vi "Keithley Log Ramp 3940 Amp.vi"(2 "Point #":i32, 3 "GPIB Data In":dbl[](array[numeric]) format="%.2e", 4 "Parameters":dbl[](array[numeric]) format="%.3e", 5 "VISA session":refnum<visa-resource-name>) -> (0 "Stop":bool, 1 "Keithley 3940 Voltage":dbl[](array[numeric]) format="%.3e")   [LabVIEW 2025]
doc: "Author: Scott Hannahs <sth@magnet.fsu.edu>\n\nThis software is licensed for use under the “MIT License\"\nCopyright (c) 2025 Scott Hannahs, sth@sth@magnet.sthnet.net\n\nPermission is hereby granted, free of charge, to any person obtaining a copy of this software and associated documentation files (the \"Software\"), to deal in the Software without restriction, including without limitation the rights to use, copy, modify, merge, publish, distribute, sublicense, and/or sell copies of the Software, and to permit persons to whom the Software is furnished to do so, subject to the following conditions: The above copyright notice and this permission notice shall be included in all copies or substantial portions of the Software.\n\nTHE SOFTWARE IS PROVIDED \"AS IS\", WITHOUT WARRANTY OF ANY KIND, EXPRESS OR IMPLIED, INCLUDING BUT NOT LIMITED TO THE WARRANTIES OF MERCHANTABILITY, FITNESS FOR A PARTICULAR PURPOSE AND NONINFRINGEMENT. IN NO EVENT SHALL THE AUTHORS OR COPYRIGHT HOLDERS BE LIABLE FOR ANY CLAIM, DAMAGES OR OTHER LIABILITY, WHETHER IN AN ACTION OF CONTRACT, TORT OR OTHERWISE, ARISING FROM, OUT OF OR IN CONNECTION WITH THE SOFTWARE OR THE USE OR OTHER DEALINGS IN THE SOFTWARE."
panel:
  out "I0":dbl format="%.3e"
  out "I":dbl format="%.3e"
  out "Delta":dbl format="%.2f"
  # "# pts/decade"
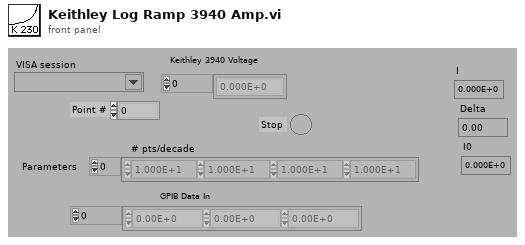
[diagram p1: front panel]
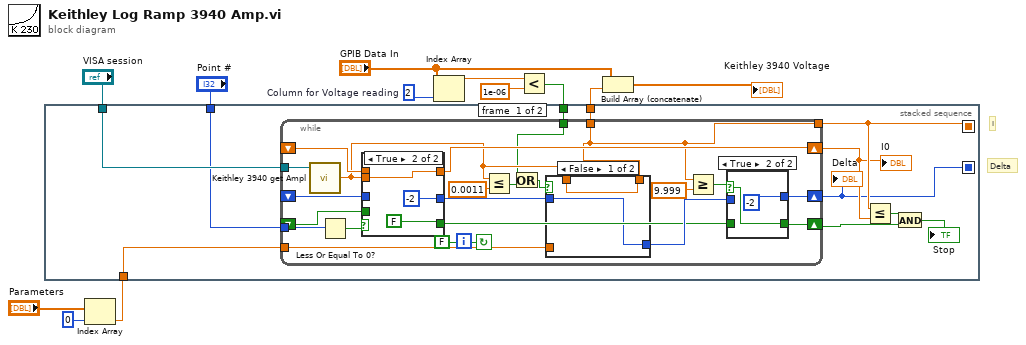
[diagram p0: block diagram]
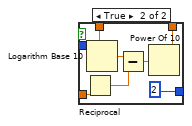
[diagram p3: hidden frame]
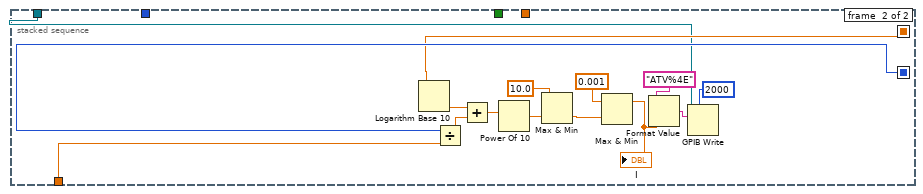
[diagram p5: hidden frame]
diagram:
  w5 = 2  # Column for Voltage reading
  # "I"
  # "Delta"
  n1 = Index Array(array="Parameters", index=0) -> (element=w9:dbl)
  n2 = Index Array(array="GPIB Data In", index=w5) -> (element=w4:dbl)
  n3 = Less?(x=w4, y=1e-06) -> (x < y?=w2:bool)
  n4 = stacked-sequence {
    seq-local: [w15 _] -> [_ w69]
    seq-local: [w18 _] -> [_ w67]
    tunnel: "VISA session" -> [w23 w65]
    tunnel: [w22 _] -> w8
    tunnel: w9 -> [w20 w70]
    tunnel: "Point #" -> [w21 _]
    tunnel: w2 -> [w13 _]
    frame #0 {
      n5 = while {
        tunnel: w13 -> [w27]
        shift-left: _ -> [w26]
        shift-right: [w30] -> w14
        tunnel: w20 -> [w33]
        tunnel: w21 -> [w34]
        tunnel: [w32] -> w18
        tunnel: [w32] -> w22
        shift-left: _ -> [w44]
        shift-right: [w36] -> w15
        tunnel: w23 -> [w38]
        shift-left: _ -> [w45]
        shift-right: [w37] -> w16
        stop <- FALSE continue-if-true
        n6 = call "Keithley 3940 get Ampl.vi"("VISA session"=w38) -> ("Amplitude"=w31:dbl)  [unwired: 1 in, 1 out]
        n7 = Less Or Equal To 0?(x=w34) -> (x <= 0?=w25:bool)
        n8 = case shown="True" w25 {
          tunnel: w45 -> [w61 _]
          tunnel: [w61 w63] -> w37
          tunnel: [w60 -2] -> w41
          tunnel: w44 -> [w60 _]
          tunnel: w31 -> [_ w63]
          tunnel: [w59 FALSE] -> w29
          tunnel: w26 -> [w59 _]
          frame False {
          }
          frame True {
          }
        }
        n9 = Less Or Equal?(x=w31, y=0.0011) -> (x <= y?=w42:bool)
        n10 = Or(x=w27, y=w42) -> (x .or. y?=w28:bool)
        n11 = case shown="False" w28 {
          tunnel: [w51 2] -> w35
          tunnel: w41 -> [w51 _]
          tunnel: w33 -> [_ w57]
          tunnel: w31 -> [w50 w56]
          tunnel: [w50 w52] -> w32
          frame False {
          }
          frame True {
            n12 = Reciprocal(x=w57) -> (1/x=w54:dbl)
            n13 = Logarithm Base 10(1:w56) -> (0:w55:dbl)
            n14 = Subtract(x=w55, y=w54) -> (x-y=w53:dbl)
            n15 = Power Of 10(x=w53) -> (10^x=w52:dbl)
          }
        }
        n16 = Greater Or Equal?(x=w32, y=9.999) -> (x >= y?=w39:bool)
        n17 = case shown="True" w39 {
          selector: w39 -> [_ w48]
          tunnel: w35 -> [w47 _]
          tunnel: [w47 -2] -> w36
          tunnel: [w46 w48] -> w30
          tunnel: w29 -> [w46 _]
          frame False {
          }
          frame True {
          }
        }
      }
      "Delta" <- w15
      "I0" <- w16
      n18 = Less Or Equal?(x=w18, y=w16) -> (x <= y?=w17:bool)
      n19 = And(x=w17, y=w14) -> (x .and. y?=→"Stop":bool)
    }
    frame #1 {
      n20 = Logarithm Base 10(1:w67) -> (0:w72:dbl)
      n21 = Divide(x=w69, y=w70) -> (x/y=w71:dbl)
      n22 = Add(x=w72, y=w71) -> (x+y=w68:dbl)
      n23 = Power Of 10(x=w68) -> (10^x=w66:dbl)
      n24 = Max & Min(x=10.0, y=w66) -> (min(x,y)=w76:dbl)  [unwired: 1 out]
      n25 = Max & Min(x=0.001, y=w76) -> (max(x,y)=w74:dbl)  [unwired: 1 out]
      "I" <- w74
      n26 = Format Value(format string="ATV%4E", value (0)=w74) -> (output string=w79:string)  [unwired: 1 in]
      n27 = GPIB Write(0:w65, 1:w79, 4:u32 2000) -> ()  [unwired: 2 in, 2 out]
    }
  }
  n28 = Build Array (concatenate)("GPIB Data In", w8) -> (→"Keithley 3940 Voltage":dbl[])
